vi "Scanner Queue - FGV.vi"(7 "FGV States":T1, 8 "error in":errorcluster, 11 "VI In":refnum<vi>) -> (0 "error out":errorcluster, 3 "queue out":refnum<queue>)   [LabVIEW 2024, in "Session Scanner.lvlib"]
uses:
  Session Scanner.lvlib
  Support/General Type Defs/FGV States.ctl
  Support/General Type Defs/Queue Message.ctl
  Support/General Type Defs/General Type Definitions.lvlib
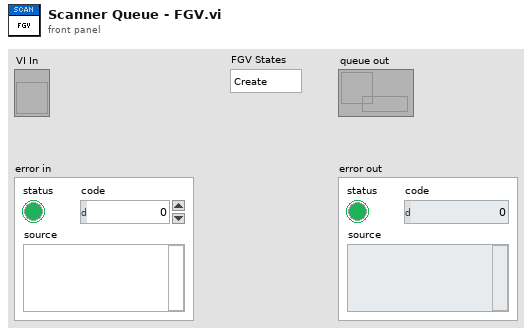
[diagram p1: front panel]
types:
  T1 = typedef "General Type Definitions.lvlib/FGV States.ctl" = enum16{"Create", "Get", "Destroy"}
  T2 = typedef "General Type Definitions.lvlib/Queue Message.ctl" = cluster{"Message":string, "Value":variant}
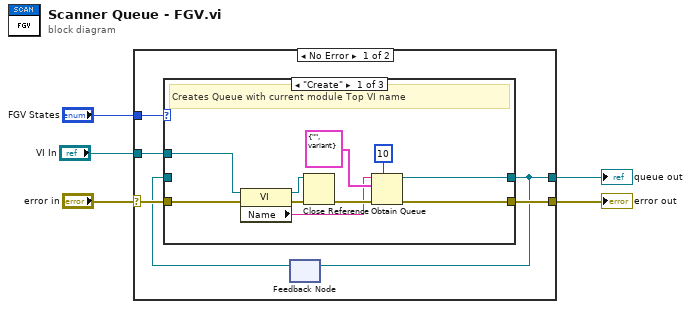
[diagram p0: block diagram]
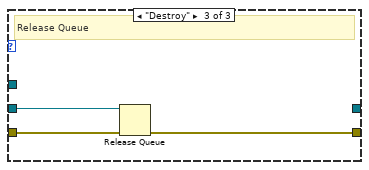
[diagram p3: hidden frame]
diagram:
  n1 = case shown="No Error" "error in" {
    selector: "error in" -> [w9 w27]
    tunnel: "FGV States" -> [w11 _]
    tunnel: [w10 w27] -> w4
    tunnel: [w8 _] -> w2
    tunnel: "VI In" -> [w6 _]
    frame No Error {
      n2 = feedback #1() -> (w7:refnum<queue>)  [unwired: 1 in]
      n3 = case shown="\"Create\"" w11 {
        tunnel: [w21 w22 w25] -> w10
        tunnel: w9 -> [w16 w22 w26]
        tunnel: [w19 w23 _] -> w8
        tunnel: w7 -> [_ w23 w24]
        tunnel: w6 -> [w14 _ _]
        frame "Create" {
          # "Creates Queue with current module Top VI name"
          n4 = property class="VI"(reference=w14, error in=w16) -> (reference out=w18:refnum<vi>, error out=w17:errorcluster, "Name"=w13:string)
          n5 = Close Reference(reference=w18, error in (no error)=w17) -> (error out=w15:errorcluster)
          n6 = Obtain Queue(max queue size (-1, unlimited)=10, name (unnamed)=w13, element data type=T2 {"Message"="", "Value"=variant}, error in (no error)=w15) -> (queue out=w19:refnum<queue>, error out=w21:errorcluster)  [unwired: 1 in, 1 out]
        }
        frame "Get", Default {
          # "Gets Queue"
        }
        frame "Destroy" {
          # "Release Queue"
          n7 = Release Queue(queue=w24, error in (no error)=w26) -> (error out=w25:errorcluster)  [unwired: 1 in, 2 out]
        }
      }
      n8 = feedback-in #1(w8) -> ()
    }
    frame Error {
    }
  }
  "error out" <- w4
  "queue out" <- w2
